vi "Instrument - Tool.vi"() -> ()   [LabVIEW 2019, in "Instrument Workspace Tool.lvlib"]
uses:
  Instrument Workspace Tool.lvlib
  NationalInstruments.VeriStand.SystemStorage
  Addon/Addon Shared/Types/Response Wait Type.ctl
  Workspace Shared/Types/State Variables.ctl
  <vilib>/NI VeriStand/Execution/Workspace/WorkspaceAPI.ctl
  <vilib>/NI VeriStand/Display Template Support/DisplayTemplateSupport.llb/enum_Display Template Handler Minimal To Workspace.ctl
  <vilib>/NI VeriStand/Display Template Support/DisplayTemplateSupport.llb/enum_Display Template Handler Minimal To Widget Msg.ctl
  <vilib>/NI/STM/TCP/TCP Connection Info.ctl
  <vilib>/NI/STM/SubVIs/MetaDataElement.ctl
  Workspace Shared/Types/CD Saved State.ctl
  <vilib>/NI VeriStand/Execution/Workspace/SystemStateEventRef.ctl
  <vilib>/NI VeriStand/Execution/Workspace/Target State Info.ctl
  <vilib>/NI VeriStand/Execution/Workspace/Target State.ctl
  <vilib>/NI VeriStand/Execution/Workspace/SystemStateRegEventRef.ctl
  Addon/Addon Shared/Types/Buffered RT Instrument Command.ctl
  <vilib>/NI VeriStand/Execution/Workspace/NI_VS Workspace ExecutionAPI.lvlib
  APIs/Host Automation API/Instrument Host Automation API.lvlib
  Addon/Addon Shared/Instrument Addon Shared.lvlib
  <vilib>/NI/STM/NI STM.lvlib
  Workspace Shared/Instrument Workspace Shared.lvlib
  NationalInstruments.VeriStand.ClientAPI
panel:
  in  "Command":string
  in  "Response?":bool
  in  "Wait Type":T1
  in  "Wait Value":dbl=100.0 format="%#_p"
  out "Timed Out?":bool
  out "Error Report":errorcluster
  out "Response":string
  in  "Send":bool
  out "Device":string
  in  "NIVS.Gateway IP Address":string
  in  "NIVS.System Definition Root":refnum<k24>
  in  "NIVS.Workspace Event":refnum<event-registration>
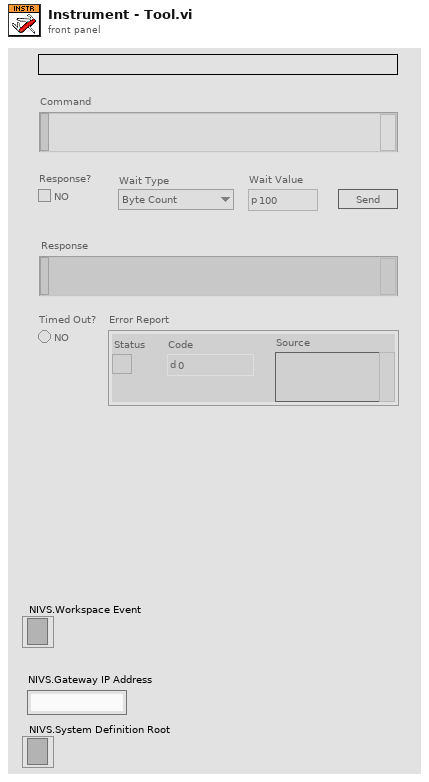
[diagram p1: front panel]
types:
  T1 = typedef "Instrument Addon Shared.lvlib/Response Wait Type.ctl" = enum16{"Byte Count", "Wait sec"}
  T2 = typedef "Instrument Workspace Shared.lvlib/State Variables.ctl" = cluster{"UI.Device":refnum<vi>, "NIVS.Workspace":T3, "NIVS.SysDefRoot":refnum<k24>, "NIVS.CachedDataRef":refnum<user-event>, "NIVS.LaunchRef":refnum<user-event>, "Addon.Comm.Info":T4, "NIVS.CachedData":T6, "NIVS.SystemStateRefs":T7, "NIVS.UserEventRefs":cluster{"WorkspaceEvent":refnum<event-registration>, "SystemChangeEventRef":T8, "LaunchRef":refnum<event-registration>}, "NIVS.Workspace Event":refnum<event-registration>, "Addon.Connected?":bool, "Mode.Tool?":bool}
  T3 = typedef "NI_VS Workspace ExecutionAPI.lvlib/WorkspaceAPI.ctl" = refnum<k24>
  T4 = typedef "NI STM.lvlib/TCP Connection Info.ctl" = cluster{"connection ID":refnum<k5>, "meta data":T5[]}
  T5 = typedef "NI STM.lvlib/MetaDataElement.ctl" = string
  T6 = typedef "Instrument Workspace Shared.lvlib/CD Saved State.ctl" = cluster{"CD Path":string, "CD IP":string}
  T7 = typedef "NI_VS Workspace ExecutionAPI.lvlib/SystemStateEventRef.ctl" = cluster{"CustDatRef":refnum<user-event>, "EvtRef":refnum<k27>, "Target State User Event":refnum<user-event>}
  T8 = typedef "NI_VS Workspace ExecutionAPI.lvlib/SystemStateRegEventRef.ctl" = refnum<event-registration>
  T9 = typedef "enum_Display Template Handler Minimal To Workspace.ctl" = cluster{"Operation":enum16{"SetCustomData", "DeleteItem"}, "Data":variant}
  T10 = typedef "Instrument Addon Shared.lvlib/Buffered RT Instrument Command.ctl" = cluster{"Command":string, "Response Expected?":bool, "Wait Type":T1, "Wait Value":dbl}
  T11 = enum8{"Enabled", "Disabled", "Disabled and Grayed Out"}
  T12 = cluster{"WorkspaceEvent":refnum<event-registration>, "SystemChangeEventRef":T8, "LaunchRef":refnum<event-registration>}
  T13 = typedef "enum_Display Template Handler Minimal To Widget Msg.ctl" = enum16{"Stop", "LaunchConfigDialog"}
  T14 = typedef "Instrument Addon Shared.lvlib/Buffered RT Instrument Request.ctl" = cluster{"Response":string, "Error":errorcluster}
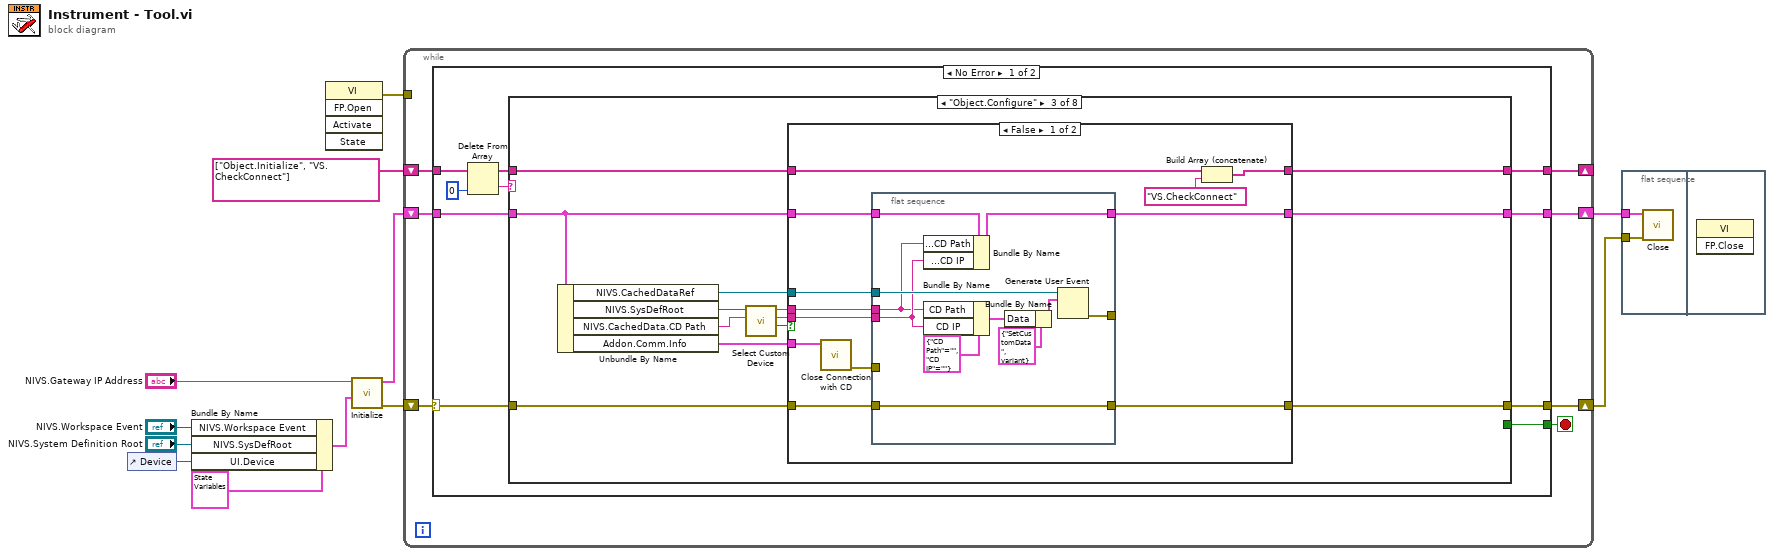
[diagram p0: block diagram]
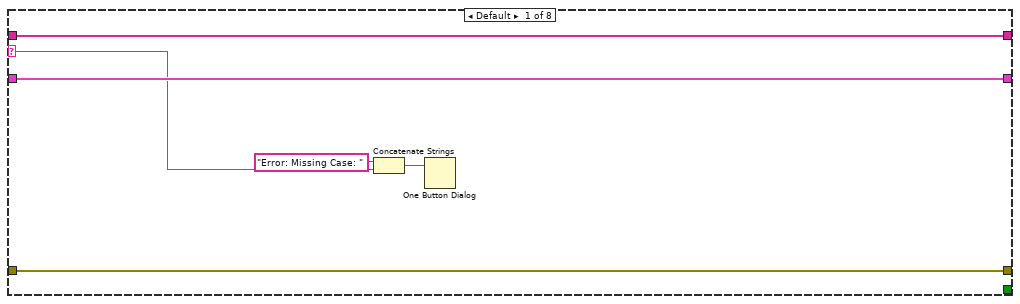
[diagram p2: hidden frame]
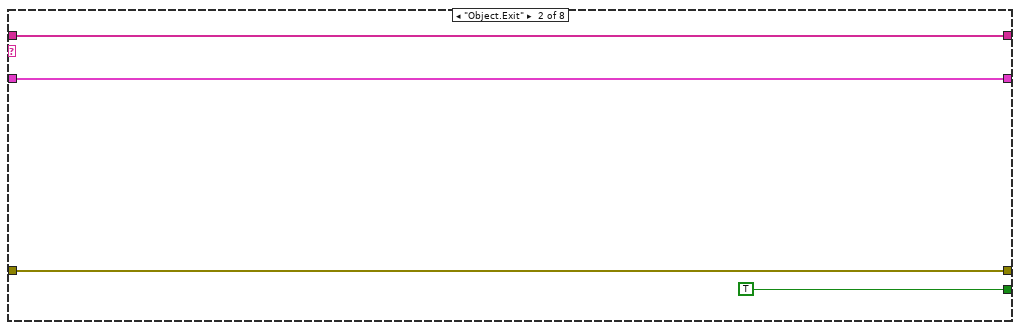
[diagram p3: hidden frame]
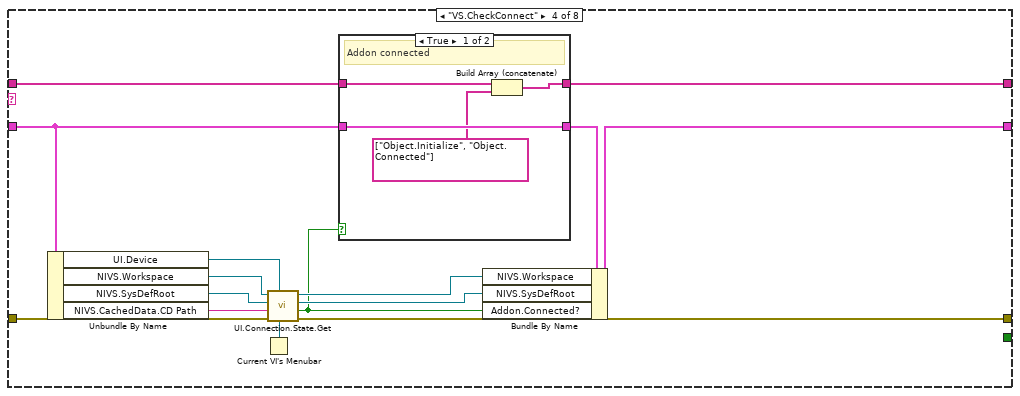
[diagram p5: hidden frame]
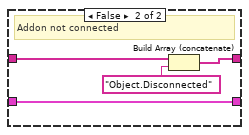
[diagram p6: hidden frame]
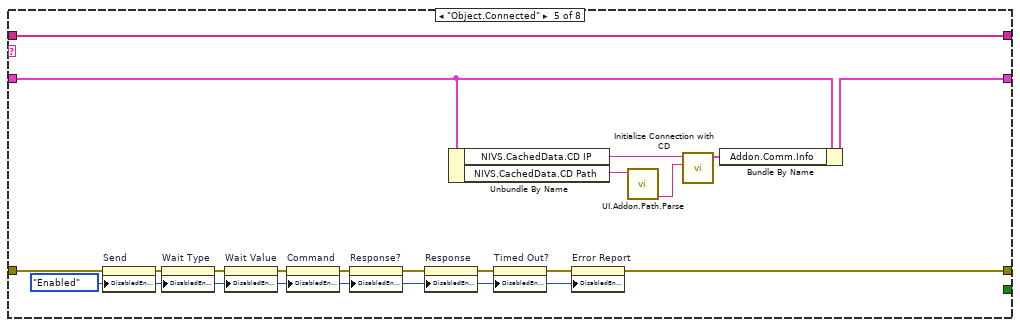
[diagram p7: hidden frame]
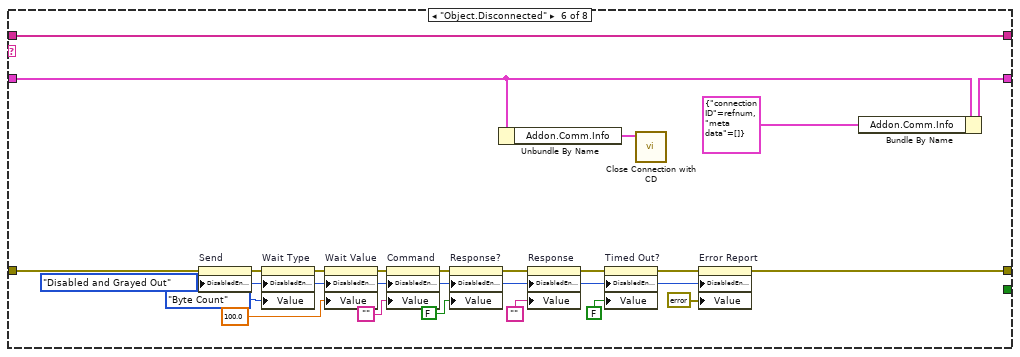
[diagram p8: hidden frame]
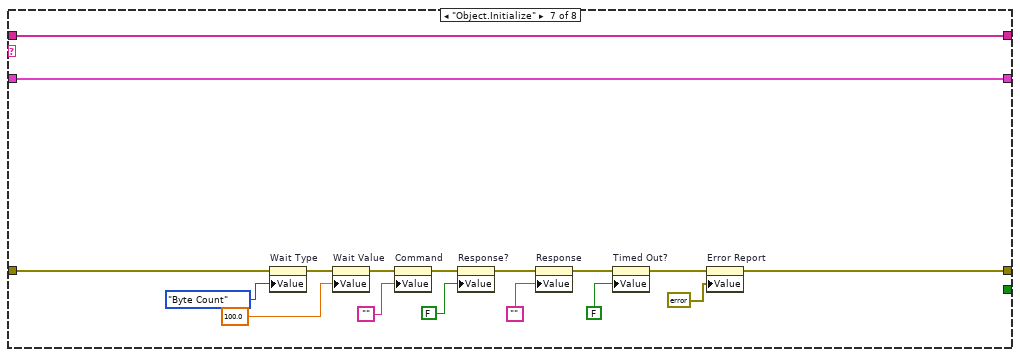
[diagram p9: hidden frame]
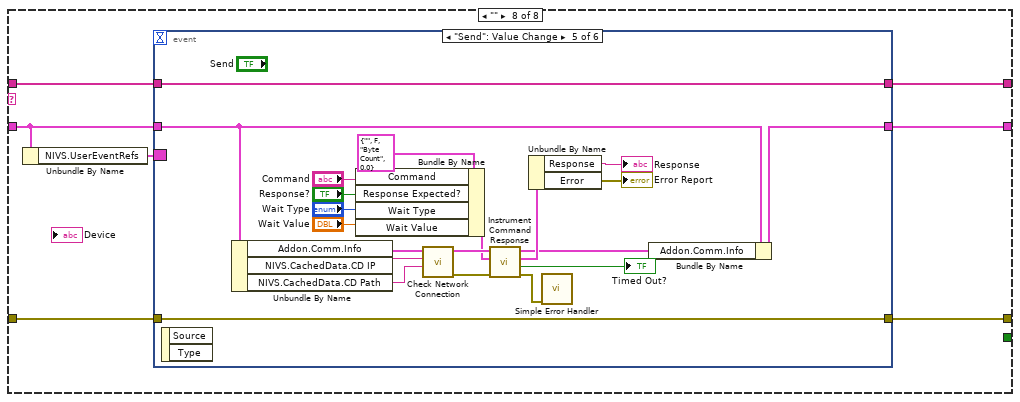
[diagram p10: hidden frame]
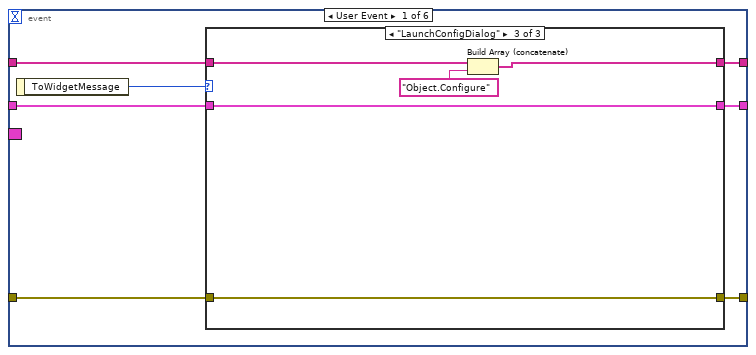
[diagram p11: hidden frame]
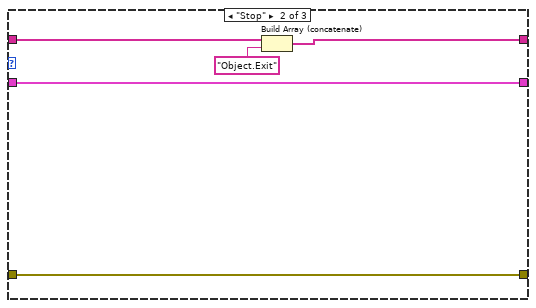
[diagram p13: hidden frame]
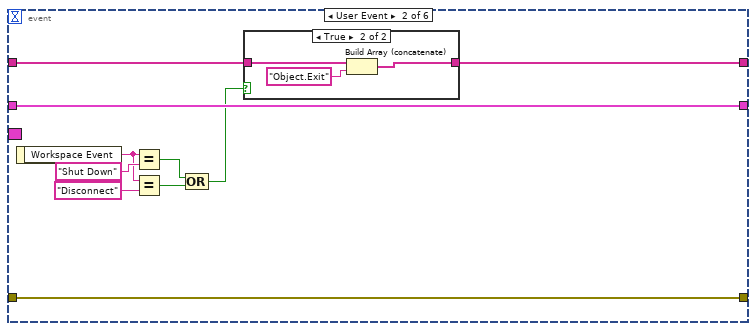
[diagram p14: hidden frame]
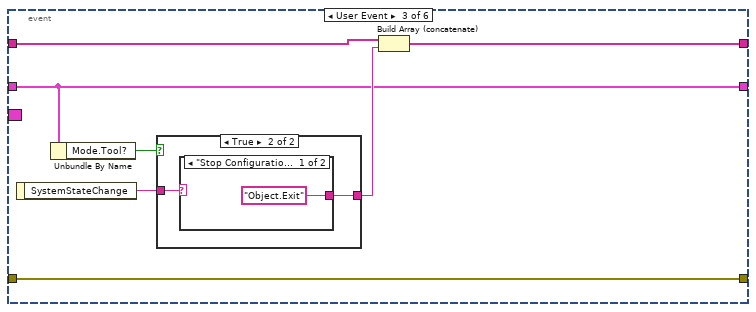
[diagram p16: hidden frame]
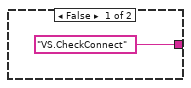
[diagram p17: hidden frame]
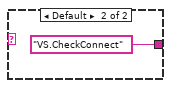
[diagram p18: hidden frame]
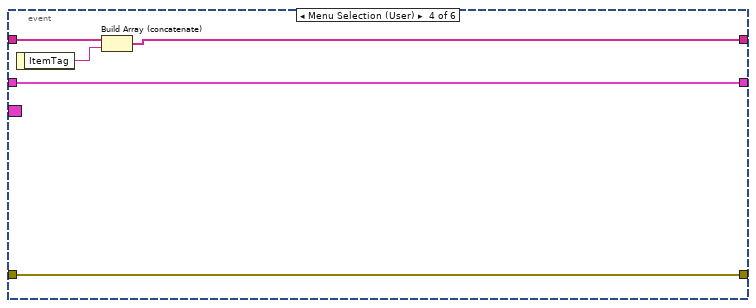
[diagram p19: hidden frame]
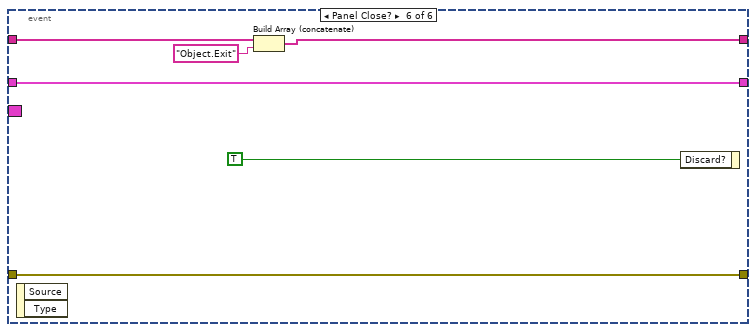
[diagram p20: hidden frame]
diagram:
  n1 = control-ref of="Device"() -> (w12:refnum<vi>)
  n2 = Bundle By Name(cluster=T2 {"UI.Device"=refnum, "NIVS.Workspace"=refnum, "NIVS.SysDefRoot"=refnum, "NIVS.CachedDataRef"=refnum, "NIVS.LaunchRef"=refnum, "Addon.Comm.Info"={"connection ID"=refnum, "meta data"=[]}, "NIVS.CachedData"={"CD Path"="", "CD IP"=""}, "NIVS.SystemStateRefs"={"CustDatRef"=refnum, "EvtRef"=refnum, "Target State User Event"=refnum}, "NIVS.UserEventRefs"={"WorkspaceEvent"=refnum, "SystemChangeEventRef"=refnum, "LaunchRef"=refnum}, "NIVS.Workspace Event"=refnum, "Addon.Connected?"=FALSE, "Mode.Tool?"=FALSE} ("State Variables in"), "NIVS.Workspace Event"="NIVS.Workspace Event", "NIVS.SysDefRoot"="NIVS.System Definition Root", "UI.Device"=w12) -> (w7:T2)
  n3 = invoke class="VI" method="FP.Open"() -> (error out=w9:errorcluster)  [unwired: 5 in, 4 out]
  n4 = call "Initialize.vi"("State Variables in"=w7, "NIVS.Gateway IP Address"="NIVS.Gateway IP Address") -> ("error out"=w6:errorcluster, "State Variables out"=w5:T2)  [unwired: 8 in]
  n5 = while {
    shift-right: [w18] -> w3
    shift-left: w6 -> [w15]
    shift-right: [w16] -> w4
    shift-left: w5 -> [w17]
    shift-right: [w13] -> _
    shift-left: string[] ["Object.Initialize", "VS.CheckConnect"] -> [w14]
    tunnel: w9 -> [_]
    stop <- w19 stop-if-true
    n6 = case shown="No Error" w15 {
      selector: w15 -> [w25 w244]
      tunnel: [w29 _] -> w19
      tunnel: [w28 w243] -> w18
      tunnel: w17 -> [w27 w247]
      tunnel: [w26 w247] -> w16
      tunnel: w14 -> [w23 w246]
      tunnel: [w20 w246] -> w13
      frame No Error {
        n7 = Delete From Array(array=w23, index=0) -> (deleted portion=w22:string, array with subset deleted=w21:string[])  [unwired: 1 in]
        n8 = case shown="\"Object.Configure\"" w22 {
          selector: w22 -> [w32 _ _ _ _ _ _ _]
          tunnel: [_ TRUE _ _ _ _ _ _] -> w29
          tunnel: [w34 w38 w46 w83 w104 w124 w146 w164] -> w28
          tunnel: w27 -> [w35 w39 w47 w92 w114 w138 w142 w162]
          tunnel: [w35 w39 w45 w91 w113 w137 w142 w161] -> w26
          tunnel: w25 -> [w34 w38 w48 w84 w118 w119 w141 w160]
          tunnel: w21 -> [w33 w37 w41 w90 w117 w140 w157 w158]
          tunnel: [w33 w37 w40 w89 w117 w140 w157 w159] -> w20
          frame Default {
            n9 = Concatenate Strings("Error: Missing Case: " ("string"), w32) -> (w31:string)
            n10 = One Button Dialog(message=w31) -> ()  [unwired: 1 in, 1 out]
          }
          frame "Object.Exit" {
          }
          frame "Object.Configure" {
            n11 = Unbundle By Name(w47) -> ("NIVS.CachedDataRef"=w51:refnum<user-event>, "NIVS.SysDefRoot"=w52:refnum<k24>, "NIVS.CachedData.CD Path"=w49:string, "Addon.Comm.Info"=w50:T4)
            n12 = call "Select Custom Device.vi"("CD Path"=w49, "NIVS.System Definition Root"=w52) -> ("Cancelled?"=w44:bool, "IP Address"=w43:string, "Cached Addon Path"=w42:string)  [unwired: 7 in]
            n13 = case shown="False" w44 {
              tunnel: w51 -> [w64 _]
              tunnel: w43 -> [w62 _]
              tunnel: w42 -> [w63 _]
              tunnel: w50 -> [w61 _]
              tunnel: [w59 w78] -> w45
              tunnel: w47 -> [w58 w78]
              tunnel: [w56 w77] -> w46
              tunnel: w48 -> [w57 w77]
              tunnel: w41 -> [w55 w76]
              tunnel: [w53 w76] -> w40
              frame False {
                n14 = call "Close Connection with CD.vi"("Comm.Info"=w61) -> ("error out"=w60:errorcluster)  [unwired: 10 in]
                n15 = flat-sequence {
                  tunnel: w64 -> [w75]
                  tunnel: w63 -> [w66]
                  tunnel: w62 -> [w69]
                  tunnel: w60 -> [_]
                  tunnel: [w71] -> w59
                  tunnel: w58 -> [w72]
                  tunnel: [w67] -> _
                  tunnel: w57 -> [w65]
                  tunnel: [w65] -> w56
                  frame #0 {
                    n16 = Bundle By Name(cluster=w72, "NIVS.CachedData.CD Path"=w66, "NIVS.CachedData.CD IP"=w69) -> (w71:T2)
                    n17 = Bundle By Name(cluster=T6 {"CD Path"="", "CD IP"=""}, "CD Path"=w66, "CD IP"=w69) -> (w68:T6)
                    n18 = Bundle By Name(cluster=T9 {"Operation"=enum."SetCustomData", "Data"=variant} ("event data"), "Data"=w68) -> (w73:T9)
                    n19 = Generate User Event(user event=w75, event data cluster=w73) -> (error out=w67:errorcluster)  [unwired: 2 in, 1 out]
                  }
                }
                n20 = Build Array (concatenate)(w55, "VS.CheckConnect") -> (w53:string[])
              }
              frame True {
              }
            }
          }
          frame "VS.CheckConnect" {
            n21 = Unbundle By Name(w92) -> ("UI.Device"=w86:refnum<vi>, "NIVS.Workspace"=w88:T3, "NIVS.SysDefRoot"=w87:refnum<k24>, "NIVS.CachedData.CD Path"=w85:string)
            n22 = Current VI's Menubar() -> (w79:refnum<k9>)
            n23 = call "UI.Connection.State.Get.vi"("Menu Ref"=w79, "Name Ref"=w86, "error in (no error)"=w84, "Addon Path in"=w85, "NIVS.System Definition Root in"=w87, "NIVS.Workspace Ref in"=w88) -> ("error out"=w83:errorcluster, "Addon Connected?"=w80:bool, "NIVS.System Definition Root out"=w81:refnum<k24>, "NIVS.Workspace Ref out"=w82:T3)  [unwired: 2 in]
            n24 = case shown="True" w80 {
              tunnel: [w97 w101] -> w89
              tunnel: [w96 w99] -> w93
              tunnel: w92 -> [w96 w99]
              tunnel: w90 -> [w95 w98]
              frame True {
                # "Addon connected"
                n25 = Build Array (concatenate)(w95, string[] ["Object.Initialize", "Object.Connected"]) -> (w97:string[])
              }
              frame False {
                # "Addon not connected"
                n26 = Build Array (concatenate)(w98, "Object.Disconnected") -> (w101:string[])
              }
            }
            n27 = Bundle By Name(cluster=w93, "NIVS.Workspace"=w82, "NIVS.SysDefRoot"=w81, "Addon.Connected?"=w80) -> (w91:T2)
          }
          frame "Object.Connected" {
            w105 = T11."Enabled" ("Disabled")
            n28 = property on="Send" class="Bool"(error in=w118, "DisabledEnum"=w105) -> (error out=w109:errorcluster)  [unwired: 1 in, 1 out]
            n29 = property on="Wait Type" class="Enum (strict)"(error in=w109, "DisabledEnum"=w105) -> (error out=w112:errorcluster)  [unwired: 1 in, 1 out]
            n30 = property on="Wait Value" class="DigNum (strict)"(error in=w112, "DisabledEnum"=w105) -> (error out=w111:errorcluster)  [unwired: 1 in, 1 out]
            n31 = property on="Command" class="Str"(error in=w111, "DisabledEnum"=w105) -> (error out=w110:errorcluster)  [unwired: 1 in, 1 out]
            n32 = property on="Response?" class="Bool (strict)"(error in=w110, "DisabledEnum"=w105) -> (error out=w106:errorcluster)  [unwired: 1 in, 1 out]
            n33 = property on="Response" class="Str"(error in=w106, "DisabledEnum"=w105) -> (error out=w107:errorcluster)  [unwired: 1 in, 1 out]
            n34 = Unbundle By Name(w114) -> ("NIVS.CachedData.CD IP"=w116:string, "NIVS.CachedData.CD Path"=w103:string)
            n35 = property on="Timed Out?" class="Bool (strict)"(error in=w107, "DisabledEnum"=w105) -> (error out=w108:errorcluster)  [unwired: 1 in, 1 out]
            n36 = property on="Error Report" class="Clust (strict)"(error in=w108, "DisabledEnum"=w105) -> (error out=w104:errorcluster)  [unwired: 1 in, 1 out]
            n37 = call "UI.Addon.Path.Parse.vi"("Cached Addon Path"=w103) -> ("Addon Name"=w102:string)  [unwired: 6 in, 4 out]
            n38 = call "Initialize Connection with CD.vi"("TCP Service"=w102, "IP Address"=w116) -> ("connection info out"=w115:T4)  [unwired: 8 in, 1 out]
            n39 = Bundle By Name(cluster=w114, "Addon.Comm.Info"=w115) -> (w113:T2)
          }
          frame "Object.Disconnected" {
            w123 = T11."Disabled and Grayed Out" ("Disabled")
            n40 = property on="Send" class="Bool"(error in=w119, "DisabledEnum"=w123) -> (error out=w133:errorcluster)  [unwired: 1 in, 1 out]
            n41 = property on="Wait Type" class="Enum (strict)"(error in=w133, "DisabledEnum"=w123, "Value"=Response_Wait_Type."Byte Count" ("Wait Type")) -> (error out=w136:errorcluster)  [unwired: 1 in, 1 out]
            n42 = property on="Wait Value" class="DigNum (strict)"(error in=w136, "DisabledEnum"=w123, "Value"=100.0 ("Wait Value")) -> (error out=w135:errorcluster)  [unwired: 1 in, 1 out]
            n43 = property on="Command" class="Str"(error in=w135, "DisabledEnum"=w123, "Value"="") -> (error out=w134:errorcluster)  [unwired: 1 in, 1 out]
            n44 = property on="Response?" class="Bool (strict)"(error in=w134, "DisabledEnum"=w123, "Value"=FALSE ("Response?")) -> (error out=w125:errorcluster)  [unwired: 1 in, 1 out]
            n45 = Unbundle By Name(w138) -> ("Addon.Comm.Info"=w139:T4)
            n46 = property on="Response" class="Str"(error in=w125, "DisabledEnum"=w123, "Value"="") -> (error out=w126:errorcluster)  [unwired: 1 in, 1 out]
            n47 = property on="Timed Out?" class="Bool (strict)"(error in=w126, "DisabledEnum"=w123, "Value"=FALSE ("Response?")) -> (error out=w127:errorcluster)  [unwired: 1 in, 1 out]
            n48 = call "Close Connection with CD.vi"("Comm.Info"=w139) -> ()  [unwired: 10 in, 1 out]
            n49 = property on="Error Report" class="Clust (strict)"(error in=w127, "DisabledEnum"=w123, "Value"=errorcluster {"Status"=FALSE, "Code"=0, "Source"=""} ("Error Report")) -> (error out=w124:errorcluster)  [unwired: 1 in, 1 out]
            n50 = Bundle By Name(cluster=w138, "Addon.Comm.Info"=T4 {"connection ID"=refnum, "meta data"=[]} ("connection info")) -> (w137:T2)
          }
          frame "Object.Initialize" {
            n51 = property on="Wait Type" class="Enum (strict)"(error in=w141, "Value"=Response_Wait_Type."Byte Count" ("Wait Type")) -> (error out=w156:errorcluster)  [unwired: 1 in, 1 out]
            n52 = property on="Wait Value" class="DigNum (strict)"(error in=w156, "Value"=100.0 ("Wait Value")) -> (error out=w155:errorcluster)  [unwired: 1 in, 1 out]
            n53 = property on="Command" class="Str"(error in=w155, "Value"="") -> (error out=w154:errorcluster)  [unwired: 1 in, 1 out]
            n54 = property on="Response?" class="Bool (strict)"(error in=w154, "Value"=FALSE ("Response?")) -> (error out=w147:errorcluster)  [unwired: 1 in, 1 out]
            n55 = property on="Response" class="Str"(error in=w147, "Value"="") -> (error out=w148:errorcluster)  [unwired: 1 in, 1 out]
            n56 = property on="Timed Out?" class="Bool (strict)"(error in=w148, "Value"=FALSE ("Response?")) -> (error out=w149:errorcluster)  [unwired: 1 in, 1 out]
            n57 = property on="Error Report" class="Clust (strict)"(error in=w149, "Value"=errorcluster {"Status"=FALSE, "Code"=0, "Source"=""} ("Error Report")) -> (error out=w146:errorcluster)  [unwired: 1 in, 1 out]
          }
          frame "" {
            n58 = Unbundle By Name(w162) -> ("NIVS.UserEventRefs"=w163:T12)
            n59 = event shown="[4] \"Send\": Value Change" {
              selector: w163 -> [_ _ _ _ _ _]
              dyn-events: _ -> [_ _ _ _ _ _]
              timeout: _ -> [_ _ _ _ _ _]
              tunnel: [w170 w190 w200 w212 w219 w242] -> w161
              tunnel: w160 -> [w167 w185 w203 w211 w218 w241]
              tunnel: [w168 w185 w203 w211 w218 w241] -> w164
              tunnel: w162 -> [w169 w190 w200 w212 w220 w242]
              tunnel: [w166 w188 w204 w213 w217 w239] -> w159
              tunnel: w158 -> [w165 w187 w205 w215 w217 w238]
              event User Event {
                n60 = event-data() -> ("ToWidgetMessage"=w171:T13)  [unwired: 1 out]
                n61 = case shown="\"LaunchConfigDialog\"" w171 {
                  tunnel: [w174 w179 w184] -> w170
                  tunnel: w169 -> [w174 w179 w184]
                  tunnel: [w173 w178 w183] -> w168
                  tunnel: w167 -> [w173 w178 w183]
                  tunnel: [w172 w176 w182] -> w166
                  tunnel: w165 -> [w172 w175 w181]
                  frame Default {
                  }
                  frame "Stop" {
                    n62 = Build Array (concatenate)(w175, "Object.Exit") -> (w176:string[])
                  }
                  frame "LaunchConfigDialog" {
                    n63 = Build Array (concatenate)(w181, "Object.Configure") -> (w182:string[])
                  }
                }
              }
              event User Event {
                n64 = event-data() -> ("Workspace Event"=w186:string)  [unwired: 1 out]
                n65 = Equal?(x=w186, y="Shut Down") -> (x = y?=w191:bool)
                n66 = Equal?(x=w186, y="Disconnect") -> (x = y?=w192:bool)
                n67 = Compound Arithmetic op=OR(w191, w192) -> (w189:bool)
                n68 = case shown="True" w189 {
                  tunnel: [w195 w197] -> w188
                  tunnel: w187 -> [w195 w196]
                  frame False {
                  }
                  frame True {
                    n69 = Build Array (concatenate)(w196, "Object.Exit") -> (w197:string[])
                  }
                }
              }
              event User Event {
                n70 = event-data() -> ("SystemStateChange"=w202:string)  [unwired: 1 out]
                n71 = Unbundle By Name(w200) -> ("Mode.Tool?"=w199:bool)
                n72 = case shown="True" w199 {
                  tunnel: ["VS.CheckConnect" w208] -> w201
                  tunnel: w202 -> [_ w207]
                  frame False {
                  }
                  frame True {
                    n73 = case shown="\"Stop Configuration\"" w207 {
                      tunnel: ["Object.Exit" "VS.CheckConnect"] -> w208
                      frame "Stop Configuration" {
                      }
                      frame Default {
                      }
                    }
                  }
                }
                n74 = Build Array (concatenate)(w205, w201) -> (w204:string[])
              }
              event Menu Selection (User) {
                n75 = event-data() -> ("ItemTag"=w214:string)  [unwired: 1 out]
                n76 = Build Array (concatenate)(w215, w214) -> (w213:string[])
              }
              event "Send": Value Change {
                n77 = event-data() -> ()  [unwired: 3 out]
                n78 = Unbundle By Name(w220) -> ("Addon.Comm.Info"=w222:T4, "NIVS.CachedData.CD IP"=w236:string, "NIVS.CachedData.CD Path"=w235:string)
                n79 = Bundle By Name(cluster=T10 {"Command"="", "Response Expected?"=FALSE, "Wait Type"=enum."Byte Count", "Wait Value"=0.0} ("Command Parameters"), "Command"="Command", "Response Expected?"="Response?", "Wait Type"="Wait Type", "Wait Value"="Wait Value") -> (w228:T10)
                n80 = call "Check Network Connection.vi"("CD Path"=w235, "IP Address"=w236, "Comm.Info"=w222) -> ("error out"=w233:errorcluster, "Comm.Info"=w234:T4)  [unwired: 7 in]
                n81 = call "Instrument Command Response.vi"("error in (no error)"=w233, "Command Parameters"=w228, "Comm.Info"=w234) -> ("error out"=w224:errorcluster, "Timed Out?"=→"Timed Out?":bool, "Response"=w226:T14, "Comm.Info"=w221:T4)  [unwired: 5 in]
                n82 = Unbundle By Name(w226) -> ("Response"=→"Response":string, "Error"=→"Error Report":errorcluster)
                n83 = call <vilib>:"Simple Error Handler.vi"("error in (no error)"=w224) -> ()  [unwired: 4 in, 5 out]
                n84 = Bundle By Name(cluster=w220, "Addon.Comm.Info"=w221) -> (w219:T2)
              }
              event Panel Close? {
                n85 = event-data() -> ()  [unwired: 3 out]
                n86 = Build Array (concatenate)(w238, "Object.Exit") -> (w239:string[])
                n87 = event-data("Discard?"=TRUE) -> ()  [unwired: 1 in, 1 out]
              }
            }
          }
        }
      }
      frame Error {
        n88 = call <vilib>:"Simple Error Handler.vi"("error in (no error)"=w244) -> ("error out"=w245:errorcluster)  [unwired: 4 in, 4 out]
        n89 = call <vilib>:"Clear Errors.vi"("error in (no error)"=w245) -> ("error out"=w243:errorcluster)  [unwired: 5 in, 1 out]
      }
    }
  }
  n90 = flat-sequence {
    tunnel: w3 -> [w249]
    tunnel: w4 -> [w248]
    frame #0 {
      n91 = call "Close.vi"("error in (no error)"=w249, "State Variables in"=w248) -> ()  [unwired: 10 in]
    }
    frame #1 {
      n92 = invoke class="VI" method="FP.Close"() -> ()  [unwired: 3 in, 3 out]
    }
  }
